vi "player_glo.vi"() -> ()   [LabVIEW 2012]
panel:
  in  "Description":string
  in  "Album":string
  in  "Titel":string
  out "running?":bool
  in  "set zeit":bool
  in  "set-zeit":dbl
  in  "loop-wait-time":dbl=100.0
  in  "error":bool
  in  "time-string":string
  in  "stop":bool
  in  "play":bool
  in  "pause":bool
  in  "forward":bool
  in  "zeit":dbl
  in  "zeitmax":dbl
  in  "volume":dbl
  in  "balance":dbl
  in  "path":path
  out "playState":i32(ring) items=["wmppsUndefined", "wmppsStopped", "wmppsPaused", "wmppsPlaying", "wmppsScanForward", "wmppsScanReverse", "wmppsBuffering", "wmppsWaiting", "wmppsMediaEnded", "wmppsTransitioning", "wmppsReady", "wmppsReconnecting", "wmppsLast"]
  # "This is a part of the player for playing musicfiles.\nAnd it's Copyright by Aron Heinecke 2009-2012"
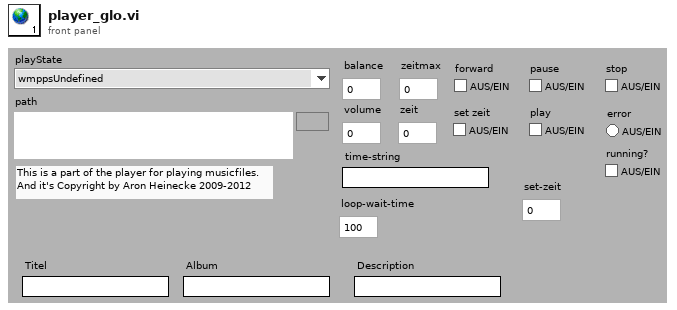
[diagram p1: front panel]
diagram:
